vi "CalibratePositions.vi"(4 "TANGO":i32, 5 "ANDORExposure":sgl, 7 "CalibStep":i32, 8 "error in (no error)":errorcluster, 9 "PosList":refnum<vi>, 11 ".NET Refnum in":refnum<k24>) -> (0 "error out":errorcluster, 1 "Elaspsed [ms]":u32, 2 "Image":T1, 3 ".NET Refnum out":refnum<k24>)   [LabVIEW 2018, in "Calibration.lvlib"]
uses:
  Calibration.lvlib
  <vilib>/vision/Image Controls.llb/IMAQ Image.ctl
  C:/Users/Familie/Documents/LabviewIX81/lib/tiff/LVTiffWriter/BitMiracle.LibTiff.NET.dll
  tiff/LVTiffWriter/BitMiracle.LibTiff.NET.dll
  ANDOR/OwnVIs/AndorOWN.lvlib
  TANGO Stage/TangoOWN.lvlib
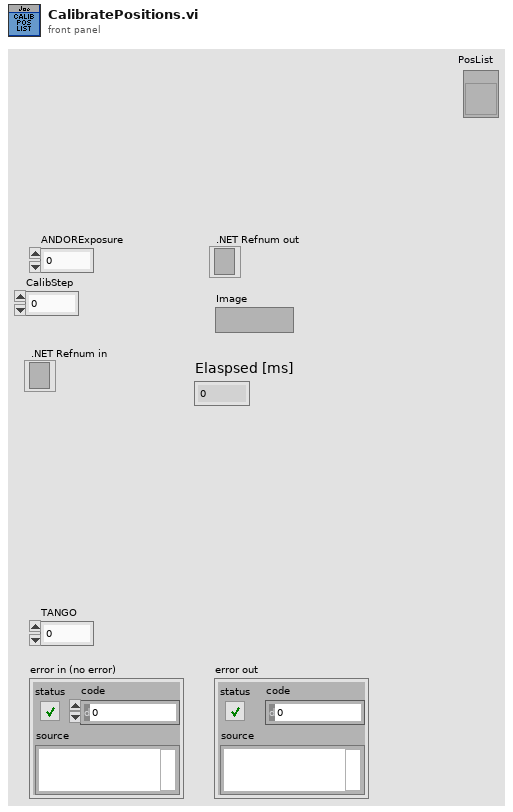
[diagram p1: front panel]
types:
  T1 = typedef "IMAQ Image.ctl" = refnum<image>
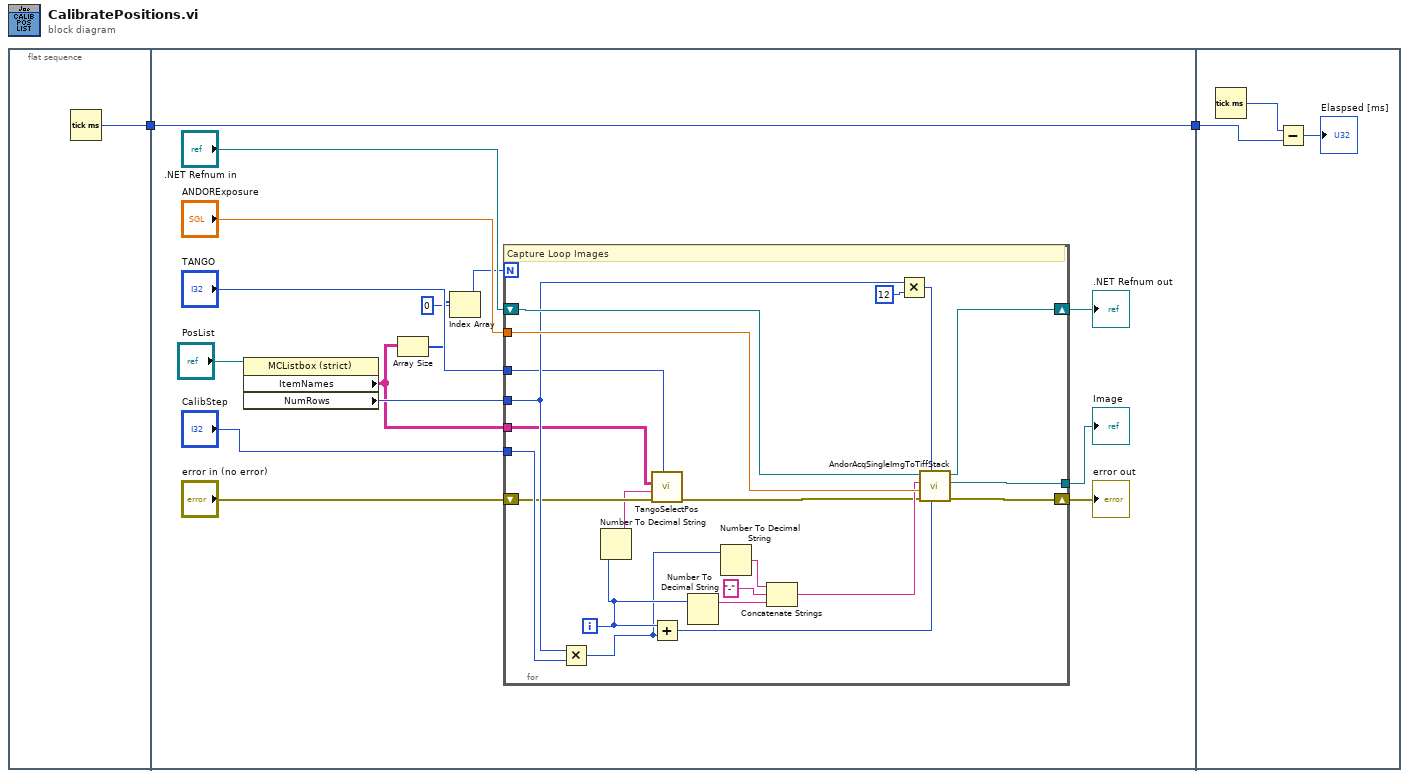
[diagram p0: block diagram]
diagram:
  n1 = flat-sequence {
    tunnel: [w3] -> w1
    tunnel: [w5] -> w2
    tunnel: w1 -> [w5]
    tunnel: w2 -> [w41]
    frame #0 {
      n2 = Tick Count (ms)() -> (millisecond timer value=w3:u32)
    }
    frame #1 {
      n3 = property on="Property Node" class="MCListbox (strict)"(reference="PosList") -> ("ItemNames"=w9:string[][], "NumRows"=w11:u32)  [unwired: 1 in, 2 out]
      n4 = Array Size(array=w9) -> (size(s)=w8:i32[])
      n5 = Index Array(array=w8, index=0) -> (element=w7:i32)
      n6 = for {
        N: w7 -> [_]
        tunnel: "ANDORExposure" -> [w38]
        tunnel: w11 -> [w26]
        shift-right: [w37] -> w14
        shift-left: ".NET Refnum in" -> [w39]
        shift-right: [w36] -> w16
        shift-left: "error in (no error)" -> [w24]
        tunnel: w9 -> [w22]
        tunnel: "TANGO" -> [w23]
        tunnel: [w34] -> w18
        tunnel: "CalibStep" -> [w27]
        i -> [w21]
        # "Capture Loop Images"
        n7 = Multiply(x=w26, y=w27) -> (x*y=w19:u32)
        n8 = Number To Decimal String(number=w21) -> (decimal integer string=w20:string)  [unwired: 1 in]
        n9 = call "TangoSelectPos.vi"("TANGO ID"=w23, "error in (no error)"=w24, "Button"=w20, "ItemNames"=w22) -> ("error out"=w25:errorcluster)  [unwired: 7 in]
        n10 = Add(x=w21, y=w19) -> (x+y=w29:u32)
        n11 = Number To Decimal String(number=w21) -> (decimal integer string=w31:string)  [unwired: 1 in]
        n12 = Number To Decimal String(number=w19) -> (decimal integer string=w28:string)  [unwired: 1 in]
        n13 = Concatenate Strings(w28, "-" ("string"), w31) -> (w35:string)
        n14 = Multiply(x=w26, y=12 ("Total Images")) -> (x*y=w33:u32)
        n15 = call "AndorAcqSingleImgToTiffStack.vi"("Image Nr"=w29, "Total Images"=w33, "error in (no error)"=w25, "Exposure"=w38, "Image Name"=w35, "TiffHandle IN"=w39) -> ("error out"=w36:errorcluster, "Image"=w34:T1, "TiffOut"=w37:refnum<k24>)  [unwired: 3 in]
      }
      "Image" <- w18
      "error out" <- w16
      ".NET Refnum out" <- w14
    }
    frame #2 {
      n16 = Tick Count (ms)() -> (millisecond timer value=w42:u32)
      n17 = Subtract(x=w42, y=w41) -> (x-y=→"Elaspsed [ms]":u32)
    }
  }
